vi "启动整机测试 (子VI).vi"() -> (0 "error out":T1={"status"=FALSE, "代码"=4, "source"=""} caption="错误输出" {"代码" items=["执行成功"=1, "执行失败，但不知道原因"=2, "命令请求条件错误"=3, "通讯超时"=4, "系统繁忙不能执行"=5, "系统故障"=6, "没有数据"=100]})   [LabVIEW 2016]
uses:
  PLC/PLC.lvlib
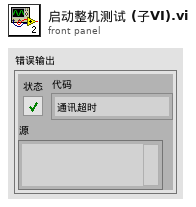
[diagram p1: front panel]
types:
  T1 = cluster{"status":bool, "代码":u16, "source":string}
  T2 = cluster{"参数启用":cluster{"氨氮":bool, "总磷":bool, "总氮":bool, "多参数":bool, "CODMn":bool, "CODcr":bool, "超标留样":bool}}
  T3 = cluster{"氨氮":bool, "总磷总氮":bool, "总氮":bool, "CODmn":bool, "CODCr":bool, "超标留样":bool, "多参数":bool}
  T4 = cluster{"自动运行启动参数":cluster{"氨氮":bool, "总磷总氮":bool, "总氮":bool, "CODmn":bool, "CODCr":bool, "超标留样":bool, "多参数":bool}}
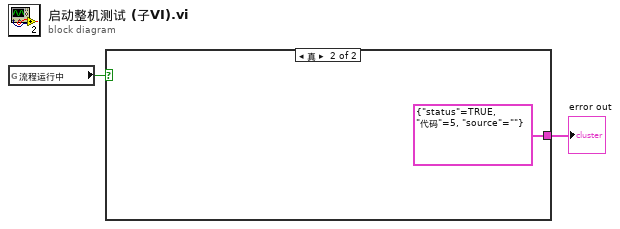
[diagram p0: block diagram]
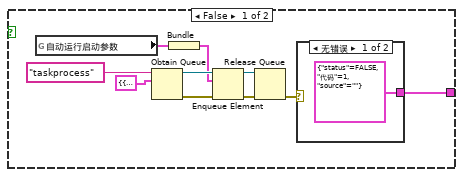
[diagram p2: hidden frame]
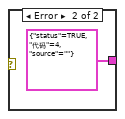
[diagram p3: hidden frame]
diagram:
  n1 = global read "采配水全局变量.vi" "流程运行中"() -> (w1:bool)
  n2 = case shown="真" w1 {
    tunnel: [w12 T1 {"status"=TRUE, "代码"=5, "source"=""} ("error out")] -> w2
    frame False {
      n3 = global read "系统设置全局变量.vi" "自动运行启动参数"() -> (w7:T3)
      n4 = Obtain Queue(name (unnamed)="taskprocess" ("名称（未命名）"), element data type=T2 {"参数启用"={"氨氮"=FALSE, "总磷"=FALSE, "总氮"=FALSE, "多参数"=FALSE, "CODMn"=FALSE, "CODcr"=FALSE, "超标留样"=FALSE}} ("参数")) -> (queue out=w9:refnum<queue>, error out=w8:errorcluster)  [unwired: 3 in, 1 out]
      n5 = Bundle("自动运行启动参数"=w7) -> (w6:T4)  [unwired: 1 in]
      n6 = Enqueue Element(queue=w9, element=w6, error in (no error)=w8) -> (queue out=w4:refnum<queue>, error out=w5:errorcluster)  [unwired: 1 in, 1 out]
      n7 = Release Queue(queue=w4, error in (no error)=w5) -> (error out=w3:errorcluster)  [unwired: 1 in, 2 out]
      n8 = case shown="无错误" w3 {
        tunnel: [T1 {"status"=FALSE, "代码"=1, "source"=""} ("error out") T1 {"status"=TRUE, "代码"=4, "source"=""} ("error out")] -> w12
        frame No Error {
        }
        frame Error {
        }
      }
    }
    frame True {
    }
  }
  "error out" <- w2
